vi "createReadDistanceFrame.vi"(8 "error in (no error)":errorcluster, 11 "DLRS1ADisplacementGauge in":refnum<class "DLRS1ADisplacementGauge.lvclass">) -> (0 "error out":errorcluster, 2 "Message":u8[](array[numeric]), 3 "DLRS1ADisplacementGauge out":refnum<class "DLRS1ADisplacementGauge.lvclass">)   [LabVIEW 2016, in "RTDLRS1ADisplacementGauge.lvlib" / "DLRS1ADisplacementGauge.lvclass"]
uses:
  DLRS1ADisplacementGauge.lvclass
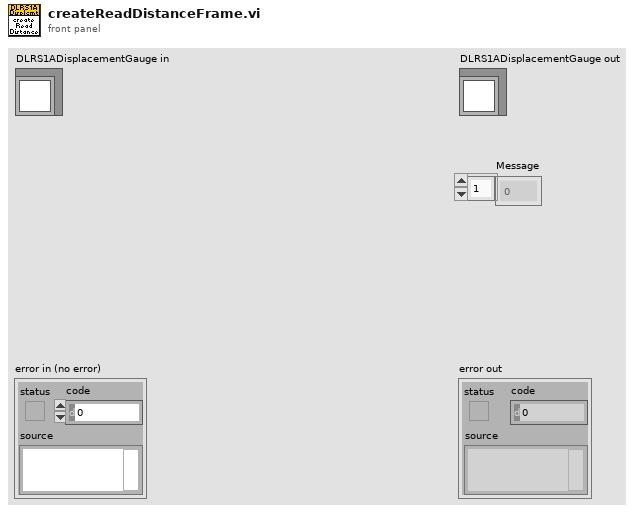
[diagram p1: front panel]
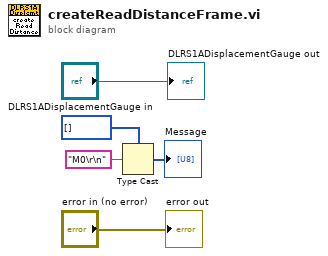
[diagram p0: block diagram]
diagram:
  n1 = Type Cast(type=u8[] [], x="M0\r\n") -> (*(type *) &x=→"Message":u8[])
  "error out" <- "error in (no error)"
  "DLRS1ADisplacementGauge out" <- "DLRS1ADisplacementGauge in"
